vi "WLAN_AMPM_DEVM_SEM.vi"() -> ()   [LabVIEW 2016]
doc: "This example illustrates how to use the RFmx and RFSG drivers and the WLAN toolkit to perform SEM and EVM measurements with or without digital predistortion (DPD) of the waveform input to the DUT. \n\nDPD is a technique to optimize the operating point of power amplifiers and other non-linear RFIC devices. Power amplifiers are much more efficient if they operate near compression. However, compressing signal amplitudes can significantly deteriorate the amplified signal's quality both, in-band (e.g., EVM increases due to non-linear distortion of the signal's I/Q constellation) and out-of-band (e.g., SEM test fails due to spectral regrowth). With DPD, the original waveform is first pre-distorted in a way that matches the non-linear effects of the RFIC device before being fed through the device. The resulting output is a much cleaner amplified and/or filtered version of the original waveform. \n\nDifferent DPD models can be used to trade off performance with computational ease, with the Lookup-Table (LUT) model the simplest and the Generalized Memory Polynomial Model (GMP) the most complex. With a LUT, the DPD algorithm achieves gain and phase linearization on average. If you want to correct for memory effects - i.e., an output sample not only depends on the current input but also previous input samples; you will notice that a specific input power value translates into a range of gain and phase values - you would use one of the memory polynomial models. For these models, several parameters such as polynomial order and memory depth are available to fine-tune the model to the DUT behavior."
uses:
  Source/SG/Typedefs/Instrument Configuration.ctl
  <instrlib>/niRFSG/niRFSG.llb/niRFSG Ref Clock Sources.ctl
  Source/Common/Local Oscillator Sharing Mode.ctl
  Source/SA/RFmxSpecAn/Typedefs/SpecAn AMPM Results.ctl
  Source/Common/SA Common Configuration.ctl
  Source/SA/RFmxWLAN/Typedefs/WLAN OFDM ModAcc Configuration.ctl
  Source/SA/RFmxWLAN/Typedefs/WLAN Standard Configuration.ctl
  Source/SA/RFmxWLAN/Typedefs/WLAN OFDM ModAcc Results.ctl
  Source/SG/Typedefs/Waveform Timing Configuration.ctl
  <instrlib>/niRFSG/niRFSG.llb/niRFSG Exported Signal Destinations.ctl
  Source/SG/Typedefs/PAEN Configuration.ctl
  Source/SA/RFmxSpecAn/Typedefs/SpecAn AMPM Configuration.ctl
  Source/Common/Waveform.ctl
  Source/SA/RFmxWLAN/Typedefs/WLAN SEM Configuration.ctl
  Source/SA/RFmxWLAN/Typedefs/WLAN SEM Results.ctl
  Source/SA/RFmxInstr/Typedefs/Instrument Configuration.ctl
  Source/Common/SA Auto Level Configuration.ctl
  <vilib>/RFmx/SpecAn/mx/RFmxSpecAn.llb/RFmxSpecAn AMPM Fetch AM to AM Trace.vi
  <vilib>/RFmx/SpecAn/mx/RFmxSpecAn.llb/RFmxSpecAn AMPM Fetch AM to PM Trace.vi
  <vilib>/RFmx/WLAN/mx/RFmxWLAN.llb/RFmxWLAN OFDMModAcc Fetch Data Constellation Trace.vi
  <vilib>/RFmx/WLAN/mx/RFmxWLAN.llb/RFmxWLAN OFDMModAcc Fetch Pilot Constellation Trace.vi
  <vilib>/RFmx/WLAN/mx/RFmxWLAN.llb/RFmxWLAN SEM Fetch Spectrum.vi
  Source/SG/SG.lvlib
  Source/SA/RFmxWLAN/RFmxWLAN.lvlib
  Source/SA/RFmxSpecAn/RFmxSpecAn.lvlib
  Source/SA/RFmxInstr/RFmxInstr.lvlib
  Source/Common/Common.lvlib
panel:
  in  "Error Tab Control":enum32{"Page 1", "Page 2"}(tab)
  out "error out":errorcluster
  in  "Display Tab Control":T1(tab)
  out "AM to PM Plot":T2(graph)
  out "AM to AM Plot":T3(graph)
  out "AMPM Measurement Results":T4 {"AM to PM Residual (deg)" format="%.2f"; "AM to AM Residual (dB)" format="%.2f"; "Mean RMS EVM (%)" format="%.2f"; "1 dB Compression Point (dBm)" format="%.2f"; "Mean Linear Gain (dB)" format="%.2f"}
  out "Constellation":cluster{sgl[], sgl[]}[](graph)
  out "OFDM ModAcc Results":T5 {"Composite Pilot RMS EVM Mean (dB)" format="%.2f"; "Composite Data RMS EVM Mean (dB)" format="%.2f"; "Composite RMS EVM Mean (dB)" format="%.2f"}
  out "WLAN SEM Results":T6 {"Upper Offset Margin Relative Power (dB)" format="%.2f"; "Upper Offset Margin Absolute Power (dBm)" format="%.2f"; "Upper Offset Margin Frequency (Hz)" format="%.3p"; "Upper Offset Margin (dB)" format="%.2f"; "Upper Offset Measurement Status" items=["Fail", "Pass"]; "Lower Offset Margin Relative Power (dB)" format="%.2f"; "Lower Offset Margin Absolute Power (dBm)" format="%.2f"; "Lower Offset Margin Frequency (Hz)" format="%.3p"; "Lower Offset Margin (dB)" format="%.2f"; "Lower Offset Measurement Status" items=["Fail", "Pass"]; "Relative Power (dB)" format="%.2f"; "Absolute Power (dBm)" format="%.2f"; "Measurement Status" items=["Fail", "Pass"]}
  out "SEM Mask":cluster{"x0":dbl, "dx":dbl, "y":sgl[]}[](graph)
  out "Reference Waveform":cluster{"t0":dbl, "dt":dbl, "y":sgl[]}(graph)
  in  "Measurement Settings Tab Control":enum32{"AM/PM", "ModAcc", "SEM"}(tab)
  in  "RFmx SpecAn AMPM Configuration":T7={"Measurement Interval (s)"=0.0001, "DUT Average Input Power (dBm)"=-20.0, "Signal Type"=0, "Averaging Enabled"=0, "Averaging Count"=10, "Reference Waveform"={"Name"="Wfm", "Data"=refnum, "Signal Bandwidth (Hz)"=0.0, "PAPR (dB)"=0.0, "Burst Length (s)"=0.0, "Sample Rate"=0.0, "Burst Start Locations"=[], "Burst Stop Locations"=[], "Idle Duration Present?"=FALSE, "Runtime Scaling"=0.0, "Script"=""}} {"Reference Waveform"."Runtime Scaling" format="%#_6p"; "Reference Waveform"."Sample Rate" format="%#_6p"; "Reference Waveform"."Burst Length (s)" format="%#_6p"; "Reference Waveform"."PAPR (dB)" format="%.2f"; "Reference Waveform"."Signal Bandwidth (Hz)" format="%#_6p"; "Averaging Enabled" items=["False", "True"]; "Signal Type" items=["Modulated", "Tones"]; "DUT Average Input Power (dBm)" format="%.2f"; "Measurement Interval (s)" format="%.2p"}
  in  "OFDM ModAcc Configuration":T9={"Acquisition Length (s)"=0.0, "Averaging Enabled"=0, "Averaging Count"=10, "Optimize Dynamic Range for EVM Enabled"=0, "Optimize Dynamic Range for EVM Margin (dB)"=0.0, "Measurement Offset (sym)"=0, "Maximum Measurement Length (sym)"=16} {"Optimize Dynamic Range for EVM Margin (dB)" format="%.2f"; "Optimize Dynamic Range for EVM Enabled" items=["False", "True"]; "Averaging Enabled" items=["False", "True"]; "Acquisition Length (s)" format="%.3p"}
  in  "WLAN SEM Configuration":T10={"Sweep Time Auto"=1, "Sweep Time (s)"=0.001, "Span Auto"=1, "Span (Hz)"=100000000.0, "Averaging Enabled"=0, "Averaging Count"=5, "Averaging Type"=0} {"Averaging Type" items=["RMS", "Log", "Scalar", "Max", "Min"]; "Averaging Enabled" items=["False", "True"]; "Span (Hz)" format="%.3p"; "Span Auto" items=["False", "True"]; "Sweep Time (s)" format="%.3p"; "Sweep Time Auto" items=["False", "True"]}
  in  "Center Frequency (Hz)":dbl=5180000000.0 format="%.6p"
  out "Resource Control":T11(tab)
  in  "RFSG Resource Name":refnum<k15>
  in  "SG Configuration":T12={"SelectedPorts"="", "Reference Clock Source"="PXI_CLK", "Carrier Frequency (Hz)"=1000000000.0, "DUT Average Input Power (dBm)"=-10.0, "External Attenuation (dB)"=0.0, "LO Sharing Mode"=enum."Automatic"}
  in  "Reference Waveform File Path":path=path "C:/Users/Public/Documents/National Instruments/RFIC Test Software/Waveforms/80211ax_80M_MCS11.tdms"
  in  "PAEN Configuration":T15={"PAEN Mode"=enum."Dynamic", "PA Enable Trigger Export Terminal"="PFI0", "PA Enable Trigger Mode"=23001, "Command Enable Time (s)"=0.0, "Command Disable Time (s)"=0.0} {"PA Enable Trigger Mode" items=["Pulse"=23000, "Toggle"=23001]; "Command Disable Time (s)" format="%#_6p"; "Command Enable Time (s)" format="%#_6p"}
  in  "Waveform Timing Configuration":T17={"Duty Cycle (%)"=50.0, "Pre-Burst Time (s)"=1e-06, "Post-Burst Time (s)"=1e-06, "Burst Start Trigger Export"="PXI_Trig0"} {"Post-Burst Time (s)" format="%#_6p"; "Pre-Burst Time (s)" format="%#_6p"; "Duty Cycle (%)" min=1.0 max=100.0 step=1.0 format="%#_2d%%"}
  in  "RFSA Resource Name":refnum<k15> caption="Resource Name"
  in  "Common Configuration":T18={"Center Frequency (Hz)"=1000000000.0, "Reference Level (dBm)"=0.0, "External Attenuation (dB)"=0.0, "Trigger Enabled"=TRUE, "Digital Trigger Source"="PXI_Trig0", "Trigger Delay (s)"=0.0, "Selected Ports"=""} {"Trigger Delay (s)" format="%.2p"; "External Attenuation (dB)" format="%.2f"; "Reference Level (dBm)" format="%.2f"; "Center Frequency (Hz)" format="%.6p"}
  in  "Instrument Configuration":T19={"LO Sharing Mode"=enum."Automatic", "Frequency Reference Source"="PXI_Clk"}
  in  "Auto Level Configuration":T20={"Enabled"=TRUE, "Measurement Interval (s)"=0.01} {"Measurement Interval (s)" min=1e-06 max=100.0 format="%.2p"}
  in  "WLAN Signal Configuration":T21={"Standard"=6, "Channel Bandwidth (Hz)"=80000000.0} {"Channel Bandwidth (Hz)" items=["5M"=5000000.0, "10M"=10000000.0, "20M"=20000000.0, "40M"=40000000.0, "80M"=80000000.0, "160M"=160000000.0]; "Standard" items=["802.11a/g", "802.11b", "802.11j", "802.11p", "802.11n", "802.11ac", "802.11ax"]}
  # "This example supports waveforms generated by the NI WLAN Generation Toolkit/Soft Front Panel and stored in the TDMS file format. Preferably, the waveform starts with one WLAN burst followed by idle time. The waveform headroom should account for the PAPR plus some margin (say 1.5 dB)."
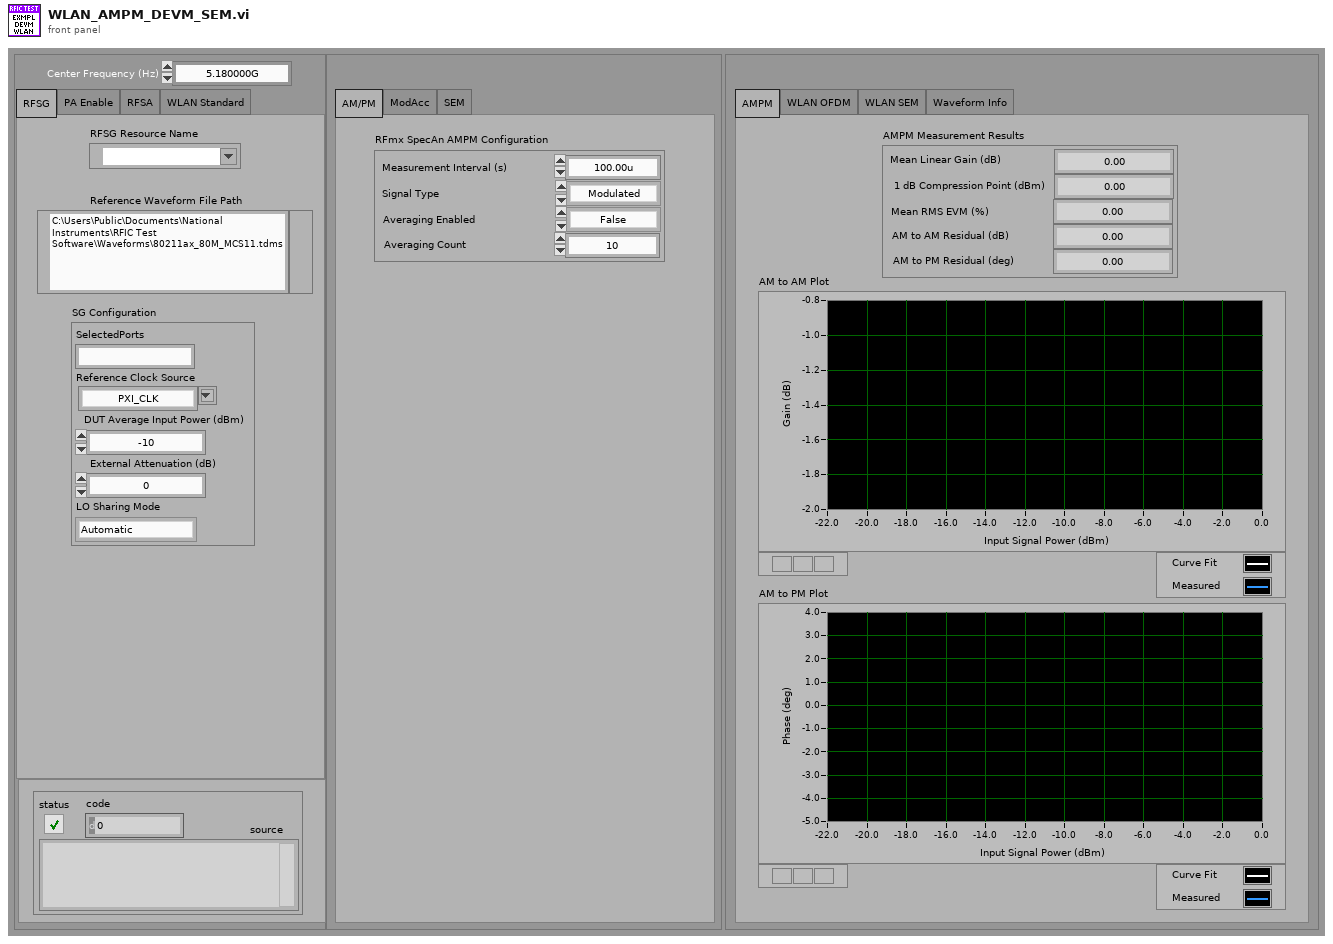
[diagram p1: front panel]
types:
  T1 = enum32{"AMPM", "WLAN OFDM", "WLAN SEM", "Waveform Info"}
  T2 = cluster{"Input Powers (dBm)":sgl[], "Curve Fit AM to PM (dB)":sgl[]}[]
  T3 = cluster{"Input Powers (dBm)":sgl[], "Curve Fit AM to AM (dB)":sgl[]}[]
  T4 = typedef "RFmxSpecAn.lvlib/SpecAn AMPM Results.ctl" = cluster{"Mean Linear Gain (dB)":dbl, "1 dB Compression Point (dBm)":dbl, "Mean RMS EVM (%)":dbl, "AM to AM Residual (dB)":dbl, "AM to PM Residual (deg)":dbl}
  T5 = typedef "RFmxWLAN.lvlib/WLAN OFDM ModAcc Results.ctl" = cluster{"Composite RMS EVM Mean (dB)":dbl, "Composite Data RMS EVM Mean (dB)":dbl, "Composite Pilot RMS EVM Mean (dB)":dbl, "Number of Symbols Used":i32}
  T6 = typedef "RFmxWLAN.lvlib/WLAN SEM Results.ctl" = cluster{"Measurement Status":i32, "Absolute Power (dBm)":dbl, "Relative Power (dB)":dbl, "Lower Offset Measurement Status":i32[], "Lower Offset Margin (dB)":dbl[], "Lower Offset Margin Frequency (Hz)":dbl[], "Lower Offset Margin Absolute Power (dBm)":dbl[], "Lower Offset Margin Relative Power (dB)":dbl[], "Upper Offset Measurement Status":i32[], "Upper Offset Margin (dB)":dbl[], "Upper Offset Margin Frequency (Hz)":dbl[], "Upper Offset Margin Absolute Power (dBm)":dbl[], "Upper Offset Margin Relative Power (dB)":dbl[]}
  T7 = typedef "RFmxSpecAn.lvlib/SpecAn AMPM Configuration.ctl" = cluster{"Measurement Interval (s)":dbl, "DUT Average Input Power (dBm)":dbl, "Signal Type":i32, "Averaging Enabled":i32, "Averaging Count":i32, "Reference Waveform":T8}
  T8 = typedef "Common.lvlib/Waveform.ctl" = cluster{"Name":string, "Data":refnum<data-value>, "Signal Bandwidth (Hz)":dbl, "PAPR (dB)":dbl, "Burst Length (s)":dbl, "Sample Rate":dbl, "Burst Start Locations":i32[], "Burst Stop Locations":i32[], "Idle Duration Present?":bool, "Runtime Scaling":dbl, "Script":string}
  T9 = typedef "RFmxWLAN.lvlib/WLAN OFDM ModAcc Configuration.ctl" = cluster{"Acquisition Length (s)":dbl, "Averaging Enabled":i32, "Averaging Count":i32, "Optimize Dynamic Range for EVM Enabled":i32, "Optimize Dynamic Range for EVM Margin (dB)":dbl, "Measurement Offset (sym)":i32, "Maximum Measurement Length (sym)":i32}
  T10 = typedef "RFmxWLAN.lvlib/WLAN SEM Configuration.ctl" = cluster{"Sweep Time Auto":i32, "Sweep Time (s)":dbl, "Span Auto":i32, "Span (Hz)":dbl, "Averaging Enabled":i32, "Averaging Count":i32, "Averaging Type":i32}
  T11 = enum32{"RFSG", "PA Enable", "RFSA", "WLAN Standard"}
  T12 = typedef "SG.lvlib/Instrument Configuration.ctl" = cluster{"SelectedPorts":string, "Reference Clock Source":T13, "Carrier Frequency (Hz)":dbl, "DUT Average Input Power (dBm)":dbl, "External Attenuation (dB)":dbl, "LO Sharing Mode":T14}
  T13 = typedef "niRFSG Ref Clock Sources.ctl" = string
  T14 = typedef "Common.lvlib/Local Oscillator Sharing Mode.ctl" = enum16{"Automatic", "None"}
  T15 = typedef "SG.lvlib/PAEN Configuration.ctl" = cluster{"PAEN Mode":enum16{"Disabled", "Static", "Dynamic"}, "PA Enable Trigger Export Terminal":T16, "PA Enable Trigger Mode":i32, "Command Enable Time (s)":dbl, "Command Disable Time (s)":dbl}
  T16 = typedef "niRFSG Exported Signal Destinations.ctl" = string
  T17 = typedef "SG.lvlib/Waveform Timing Configuration.ctl" = cluster{"Duty Cycle (%)":dbl, "Pre-Burst Time (s)":dbl, "Post-Burst Time (s)":dbl, "Burst Start Trigger Export":T16}
  T18 = typedef "Common.lvlib/SA Common Configuration.ctl" = cluster{"Center Frequency (Hz)":dbl, "Reference Level (dBm)":dbl, "External Attenuation (dB)":dbl, "Trigger Enabled":bool, "Digital Trigger Source":string, "Trigger Delay (s)":dbl, "Selected Ports":string}
  T19 = typedef "RFmxInstr.lvlib/Instrument Configuration.ctl" = cluster{"LO Sharing Mode":T14, "Frequency Reference Source":string}
  T20 = typedef "Common.lvlib/SA Auto Level Configuration.ctl" = cluster{"Enabled":bool, "Measurement Interval (s)":dbl}
  T21 = typedef "RFmxWLAN.lvlib/WLAN Standard Configuration.ctl" = cluster{"Standard":i32, "Channel Bandwidth (Hz)":dbl}
  T22 = enum16{"TXP", "PowerRamp", "DSSSModAcc", "OFDMModAcc", "SEM"}[]
  T23 = enum16{"ACP", "CCDF", "CHP", "FCnt", "Harmonics", "OBW", "SEM", "Spectrum", "Spur", "TXP", "AMPM", "DPD", "IQ", "IM", "NF", "PhaseNoise", "PAVT"}[]
  T24 = cluster{"Reference Powers (dBm)":sgl[], "Curve Fit AM to AM (dB)":sgl[]}
  T25 = cluster{"Reference Powers (dBm)":sgl[], "Measured AM to AM (dB)":sgl[]}
  T26 = cluster{"Reference Powers (dBm)":sgl[], "Curve Fit AM to PM (deg)":sgl[]}
  T27 = cluster{"Reference Powers (dBm)":sgl[], "Measured AM to PM (deg)":sgl[]}
  T28 = cluster{"Reference Powers (dBm)":sgl[], "Measured AM to AM (dB)":sgl[]}[]
  T29 = cluster{"Reference Powers (dBm)":sgl[], "Measured AM to PM (deg)":sgl[]}[]
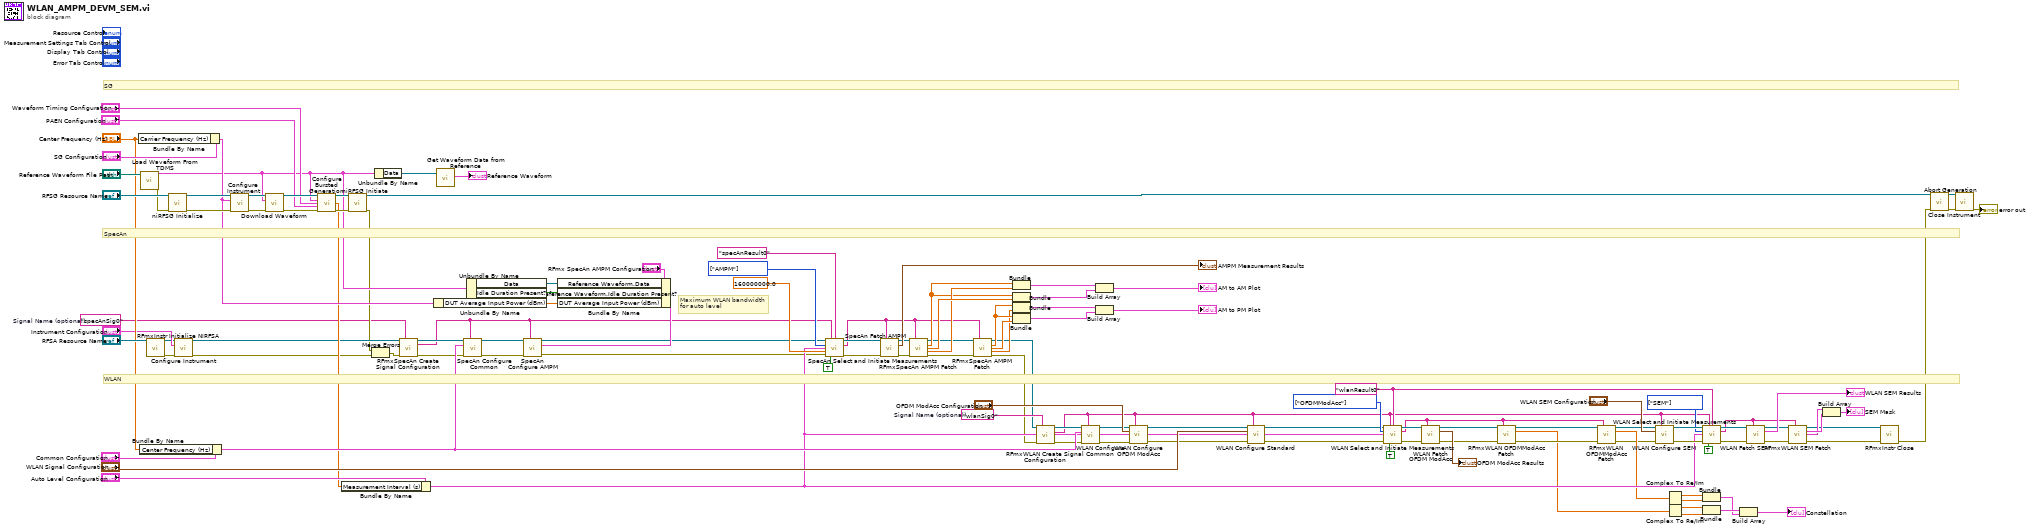
[diagram p0: block diagram]
diagram:
  w13 = "wlanResult0" ("Result Name")
  w17 = "specAnSig0"  # Signal Name (optional)
  w27 = "wlanSig0"  # Signal Name (optional)
  w47 = T22 [enum."SEM"] items=["TXP", "PowerRamp", "DSSSModAcc", "OFDMModAcc", "SEM"] ("Measurements")
  w55 = T23 [enum."AMPM"] items=["ACP", "CCDF", "CHP", "FCnt", "Harmonics", "OBW", "SEM", "Spectrum", "Spur", "TXP", "AMPM", "DPD", "IQ", "IM", "NF", "PhaseNoise", "PAVT"] ("Measurements")
  w64 = T22 [enum."OFDMModAcc"] items=["TXP", "PowerRamp", "DSSSModAcc", "OFDMModAcc", "SEM"] ("Measurements")
  # "Maximum WLAN bandwidth\nfor auto level"
  # "SpecAn"
  # "WLAN"
  # "SG"
  n1 = Bundle By Name(cluster="SG Configuration", "Carrier Frequency (Hz)"="Center Frequency (Hz)") -> (w74:T12)
  n2 = Bundle By Name(cluster="Common Configuration", "Center Frequency (Hz)"="Center Frequency (Hz)") -> (w69:T18)
  n3 = call "Load Waveform From TDMS.vi"("TDMS File Path"="Reference Waveform File Path") -> ("Waveform"=w65:T8, "error out"=w105:errorcluster)  [unwired: 13 in]
  n4 = call <vilib>:"RFmxInstr Initialize NIRFSA.vi"("Resource Name"="RFSA Resource Name") -> ("Instrument Handle Out"=w25:refnum<k21>, "error out"=w24:errorcluster)  [unwired: 12 in, 1 out]
  n5 = call <instrlib>:"niRFSG Initialize.vi"("resource name"="RFSG Resource Name", "error in"=w105) -> ("instrument handle"=w122:refnum<k15>, "error out"=w121:errorcluster)  [unwired: 12 in]
  n6 = call "Configure Instrument.vi"("Instrument Handle In"=w25, "Instrument Configuration"="Instrument Configuration", "error in (no error)"=w24) -> ("Instrument Handle Out"=w22:refnum<k21>, "error out"=w23:errorcluster)  [unwired: 11 in]
  n7 = call "Configure Instrument.vi"("RFSG Session In"=w122, "SG Configuration"=w74, "error in (no error)"=w121) -> ("RFSG Session Out"=w123:refnum<k15>, "error out"=w104:errorcluster)  [unwired: 11 in]
  n8 = call "Download Waveform.vi"("RFSG handle"=w123, "Waveform In"=w65, "error in (no error)"=w104) -> ("RFSG handle out"=w120:refnum<k15>, "error out"=w119:errorcluster)  [unwired: 11 in]
  n9 = call "Configure Bursted Generation.vi"("RFSG handle"=w120, "Waveform"=w65, "Waveform Timing Configuration"="Waveform Timing Configuration", "PAEN Configuration"="PAEN Configuration", "error in"=w119) -> ("RFSG handle out"=w106:refnum<k15>, "Generation Period (s)"=w52:dbl, "error out"=w101:errorcluster)  [unwired: 7 in, 1 out]
  n10 = Bundle By Name(cluster="Auto Level Configuration", "Measurement Interval (s)"=w52) -> (w46:T20)
  n11 = call <instrlib>:"niRFSG Initiate.vi"("instrument handle"=w106, "error in"=w101) -> ("instrument handle out"=w70:refnum<k15>, "error out"=w18:errorcluster)  [unwired: 12 in]
  n12 = Merge Errors(w18, w23) -> (w19:errorcluster)
  n13 = Unbundle By Name(w65) -> ("Data"=w67:refnum<data-value>)
  n14 = call <vilib>:"RFmxSpecAn Create Signal Configuration.vi"("Instrument Handle In"=w22, "Signal Name"=w17, "error in (no error)"=w19) -> ("Instrument Handle Out"=w20:refnum<k21>, "Selector String Out"=w16:string, "error out"=w21:errorcluster)  [unwired: 10 in]
  n15 = Unbundle By Name(w74) -> ("DUT Average Input Power (dBm)"=w71:dbl)
  n16 = call "Get Waveform Data from Reference.vi"("Waveform Data Reference"=w67) -> ("Waveform Data"=→"Reference Waveform":cluster{"t0":dbl, "dt":dbl, "y":csg[]})  [unwired: 13 in, 1 out]
  n17 = call "SpecAn Configure Common.vi"("RFmx Handle In"=w20, "Selector String"=w16, "Common Configuration"=w69, "error in (no error)"=w21) -> ("RFmx Handle Out"=w10:refnum<k21>, "error out"=w9:errorcluster)  [unwired: 10 in]
  n18 = Unbundle By Name(w65) -> ("Data"=w112:refnum<data-value>, "Idle Duration Present?"=w111:bool)
  n19 = Bundle By Name(cluster="RFmx SpecAn AMPM Configuration", "Reference Waveform.Data"=w112, "Reference Waveform.Idle Duration Present?"=w111, "DUT Average Input Power (dBm)"=w71) -> (w113:T7)
  n20 = call "SpecAn Configure AMPM.vi"("RFmx Handle In"=w10, "Selector String"=w16, "RFmx SpecAn AMPM Configuration"=w113, "error in (no error)"=w9) -> ("RFmx Handle Out"=w8:refnum<k21>, "error out"=w7:errorcluster)  [unwired: 10 in]
  n21 = call "SpecAn Select and Initiate Measurements.vi"("Instrument Handle In"=w8, "Selector String"=w16, "Result Name"="specAnResult0", "Measurements"=w55, "Auto Level Configuration"=w46, "Auto Level Bandwidth (Hz)"=160000000.0, "error in (no error)"=w7, "Enable All Traces (F)"=TRUE ("Enable All Traces")) -> ("Instrument Handle Out"=w58:refnum<k21>, "Selector String Out"=w14:string, "error out"=w57:errorcluster)  [unwired: 5 in]
  n22 = call "SpecAn Fetch AMPM.vi"("RFmx Handle In"=w58, "Selector String"=w14, "error in (no error)"=w57) -> ("RFmx Handle Out"=w85:refnum<k21>, "AMPM Results"=→"AMPM Measurement Results":T4, "error out"=w84:errorcluster)  [unwired: 10 in]
  n23 = call-poly <vilib>:"RFmxSpecAn AMPM Fetch.vi"("Instrument Handle In"=w85, "Selector String"=w14, "error in (no error)"=w84) -> ("Instrument Handle Out"=w91:refnum<k21>, "Reference Powers (dBm)"=w95:sgl[], "Measured AM to AM (dB)"=w97:sgl[], "Curve Fit AM to AM (dB)"=w96:sgl[], "error out"=w90:errorcluster)  [unwired: 8 in]
  n24 = call-poly <vilib>:"RFmxSpecAn AMPM Fetch.vi"("Instrument Handle In"=w91, "Selector String"=w14, "error in (no error)"=w90) -> ("Instrument Handle Out"=w2:refnum<k21>, "Reference Powers (dBm)"=w94:sgl[], "Measured AM to PM (deg)"=w93:sgl[], "Curve Fit AM to PM (deg)"=w92:sgl[], "error out"=w1:errorcluster)  [unwired: 8 in]
  n25 = Bundle("Reference Powers (dBm)"=w95, "Curve Fit AM to AM (dB)"=w96) -> (w89:T24)  [unwired: 1 in]
  n26 = Bundle("Reference Powers (dBm)"=w95, "Measured AM to AM (dB)"=w97) -> (w88:T25)  [unwired: 1 in]
  n27 = Bundle("Reference Powers (dBm)"=w94, "Curve Fit AM to PM (deg)"=w92) -> (w86:T26)  [unwired: 1 in]
  n28 = Bundle("Reference Powers (dBm)"=w94, "Measured AM to PM (deg)"=w93) -> (w87:T27)  [unwired: 1 in]
  n29 = call <vilib>:"RFmxWLAN Create Signal Configuration.vi"("Instrument Handle In"=w2, "Signal Name"=w27, "error in (no error)"=w1) -> ("Instrument Handle Out"=w29:refnum<k21>, "Selector String Out"=w11:string, "error out"=w28:errorcluster)  [unwired: 10 in]
  n30 = call "WLAN Configure Common.vi"("Instrument Handle In"=w29, "Selector String"=w11, "Common Configuration"=w69, "error in (no error)"=w28) -> ("Instrument Handle Out"=w73:refnum<k21>, "error out"=w72:errorcluster)  [unwired: 10 in]
  n31 = Build Array(w89, w88) -> (→"AM to AM Plot":T28)
  n32 = Build Array(w86, w87) -> (→"AM to PM Plot":T29)
  n33 = call "WLAN Configure OFDM ModAcc.vi"("Instrument Handle In"=w73, "Selector String"=w11, "OFDM ModAcc Configuration"="OFDM ModAcc Configuration", "error in (no error)"=w72) -> ("Instrument Handle Out"=w6:refnum<k21>, "error out"=w5:errorcluster)  [unwired: 10 in]
  n34 = call "WLAN Configure Standard.vi"("Instrument Handle In"=w6, "Selector String"=w11, "WLAN Standard Configuration"="WLAN Signal Configuration", "error in (no error)"=w5) -> ("Instrument Handle Out"=w63:refnum<k21>, "error out"=w62:errorcluster)  [unwired: 10 in]
  n35 = call "WLAN Select and Initiate Measurements.vi"("Instrument Handle In"=w63, "Selector String"=w11, "Result Name"=w13, "Measurements"=w64, "Auto Level Configuration"=w46, "error in (no error)"=w62, "Enable All Traces (F)"=TRUE) -> ("Instrument Handle Out"=w61:refnum<k21>, "Selector String Out"=w26:string, "error out"=w60:errorcluster)  [unwired: 6 in]
  n36 = call "WLAN Fetch OFDM ModAcc.vi"("Instrument Handle In"=w61, "Selector String"=w26, "error in (no error)"=w60) -> ("Instrument Handle Out"=w37:refnum<k21>, "OFDM ModAcc Results"=→"OFDM ModAcc Results":T5, "error out"=w36:errorcluster)  [unwired: 10 in]
  n37 = call-poly <vilib>:"RFmxWLAN OFDMModAcc Fetch.vi"("Instrument Handle In"=w37, "Selector String"=w26, "error in (no error)"=w36) -> ("Instrument Handle Out"=w35:refnum<k21>, "Data Constellation"=w31:csg[], "error out"=w34:errorcluster)  [unwired: 10 in]
  n38 = call-poly <vilib>:"RFmxWLAN OFDMModAcc Fetch.vi"("Instrument Handle In"=w35, "Selector String"=w26, "error in (no error)"=w34) -> ("Instrument Handle Out"=w32:refnum<k21>, "Pilot Constellation"=w38:csg[], "error out"=w33:errorcluster)  [unwired: 10 in]
  n39 = call "WLAN Configure SEM.vi"("Instrument Handle In"=w32, "Selector String"=w11, "WLAN SEM Configuration"="WLAN SEM Configuration", "error in (no error)"=w33) -> ("Instrument Handle Out"=w51:refnum<k21>, "error out"=w49:errorcluster)  [unwired: 10 in]
  n40 = Complex To Re/Im(x + iy=w38) -> (x=w42:sgl[], y=w41:sgl[])
  n41 = Complex To Re/Im(x + iy=w31) -> (x=w44:sgl[], y=w43:sgl[])
  n42 = Bundle(w44, w43) -> (w40:cluster{sgl[], sgl[]})  [unwired: 1 in]
  n43 = call "WLAN Select and Initiate Measurements.vi"("Instrument Handle In"=w51, "Selector String"=w11, "Result Name"=w13, "Measurements"=w47, "Auto Level Configuration"=w46, "error in (no error)"=w49, "Enable All Traces (F)"=TRUE) -> ("Instrument Handle Out"=w50:refnum<k21>, "Selector String Out"=w12:string, "error out"=w48:errorcluster)  [unwired: 6 in]
  n44 = Bundle(w42, w41) -> (w39:cluster{sgl[], sgl[]})  [unwired: 1 in]
  n45 = Build Array(w40, w39) -> (→"Constellation":cluster{sgl[], sgl[]}[])
  n46 = call "WLAN Fetch SEM.vi"("Instrument Handle In"=w50, "Selector String"=w12, "error in (no error)"=w48) -> ("Instrument Handle Out"=w79:refnum<k21>, "WLAN SEM Results"=→"WLAN SEM Results":T6, "error out"=w78:errorcluster)  [unwired: 10 in]
  n47 = call-poly <vilib>:"RFmxWLAN SEM Fetch.vi"("Instrument Handle In"=w79, "Selector String"=w12, "error in (no error)"=w78) -> ("Instrument Handle Out"=w3:refnum<k21>, "Spectrum (dBm)"=w77:cluster{"x0":dbl, "dx":dbl, "y":sgl[]}, "Composite Mask (dBm)"=w76:cluster{"x0":dbl, "dx":dbl, "y":sgl[]}, "error out"=w4:errorcluster)  [unwired: 9 in]
  n48 = Build Array(w76, w77) -> (→"SEM Mask":cluster{"x0":dbl, "dx":dbl, "y":sgl[]}[])
  n49 = call <vilib>:"RFmxInstr Close.vi"("Instrument Handle In"=w3, "error in (no error)"=w4) -> ("error out"=w115:errorcluster)  [unwired: 13 in]
  n50 = call "Abort Generation.vi"("RFSG handle"=w70, "error in (no error)"=w115) -> ("RFSG handle out"=w124:refnum<k15>, "error out"=w125:errorcluster)  [unwired: 12 in]
  n51 = call "Close Instrument.vi"("RFSG Handle"=w124, "error in (no error)"=w125) -> ("error out"=→"error out":errorcluster)  [unwired: 13 in]
